vi "AB_Engine_Check_For_Dep_FileTypes.vi"(1 "destination in":i32, 2 "File":T2, 4 "depedentDestinationIndex":i32) -> (6 "destination out":i32)   [LabVIEW 2020]
uses:
  <vilib>/Utility/lvfile.llb/LVFileType.ctl
  <vilib>/Utility/lvfile.llb/NI_FileType.lvlib
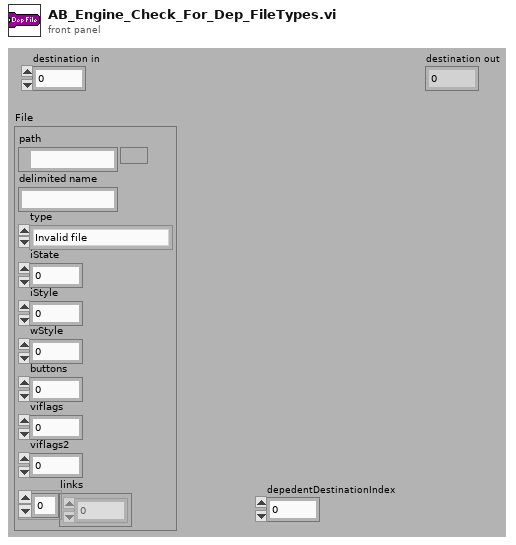
[diagram p1: front panel]
types:
  T1 = typedef "NI_FileType.lvlib/LVFileType.ctl" = enum32{"Invalid file", "Unknown type", "Instrument", "Control", "Polymorphic VI", "Project", "Library", "LVClass", "XControl", "XNode", "Shared library", ".NET assembly", "ActiveX interface", "CIN", "Run-time menu", "Palette menu", "Help file", "LLB", "XNode Edit Dependency", "Class Private Data Control", "Statechart", "MathScript .m file", "Ladder Diagram", "LVLibp", "XNode Build Dependency"}
  T2 = cluster{"path":path, "delimited name":string, "type":T1, "iState":u32, "iStyle":u16, "wStyle":u16, "buttons":u16, "viflags":u32, "viflags2":u32, "links":u32[]}
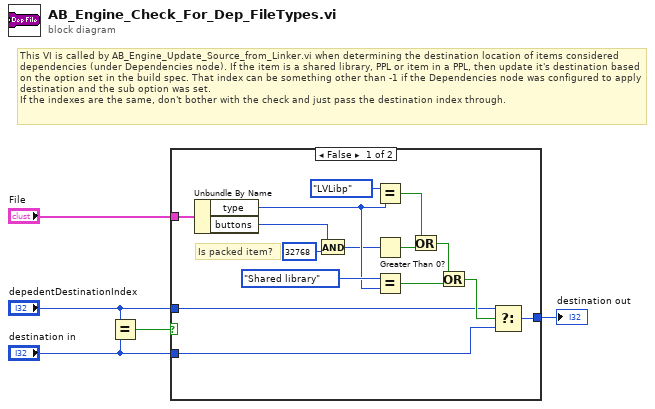
[diagram p0: block diagram]
diagram:
  # "This VI is called by AB_Engine_Update_Source_from_Linker.vi when determining the destination location of items considered dependencies (under Dependencies node). If the item is a shared library, PPL or item in a PPL, then update it's destination based on the option set in the build spec. That index can be something other than -1 if the Dependencies node was configured to apply destination and the sub option was set.\nIf the indexes are the same, don't bother with the check and just pass the destination index through."
  n1 = Equal?(x="depedentDestinationIndex", y="destination in") -> (x = y?=w1:bool)
  n2 = case shown="False" w1 {
    tunnel: "File" -> [w20 _]
    tunnel: [w8 w21] -> w4
    tunnel: "depedentDestinationIndex" -> [w7 _]
    tunnel: "destination in" -> [w6 w21]
    frame False {
      # "Is packed item?"
      n3 = Unbundle By Name(w20) -> ("type"=w17:T1, "buttons"=w15:u16)
      n4 = And(x=w15, y=u16 32768) -> (x .and. y?=w14:u16)
      n5 = Equal?(x=LVFileType."LVLibp", y=w17) -> (x = y?=w13:bool)
      n6 = Greater Than 0?(x=w14) -> (x > 0?=w12:bool)
      n7 = Equal?(x=LVFileType."Shared library", y=w17) -> (x = y?=w10:bool)
      n8 = Or(x=w13, y=w12) -> (x .or. y?=w11:bool)
      n9 = Or(x=w11, y=w10) -> (x .or. y?=w9:bool)
      n10 = Select(t=w7, s=w9, f=w6) -> (s? t:f=w8:i32)
    }
    frame True {
    }
  }
  "destination out" <- w4
